vi "error sum.vi"(1 "dead time error":dbl, 2 "Tails error":dbl, 3 "Current error":dbl) -> (0 "Delta stable current value":dbl)   [LabVIEW 2016]
doc: "This is the sum of the errors that make up the internal error. It is refered to in ursula as (delta q/q)^2"
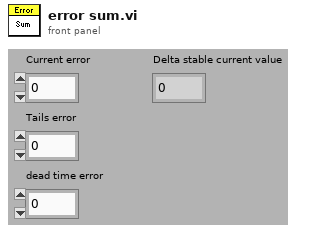
[diagram p1: front panel]
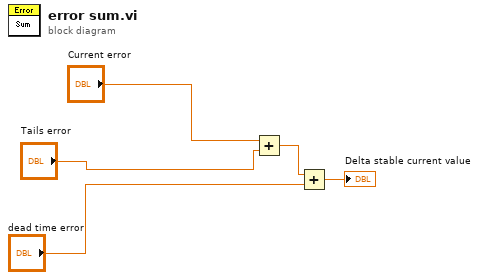
[diagram p0: block diagram]
diagram:
  n1 = Add(x="Current error", y="Tails error") -> (x+y=w3:dbl)
  n2 = Add(x=w3, y="dead time error") -> (x+y=→"Delta stable current value":dbl)
